vi "Get Ack.vi"(8 "Error In":errorcluster, 11 "connection ID":refnum<k16>) -> (0 "Error Out":errorcluster, 2 "Ack status":bool, 3 "connection ID out":refnum<k16>)   [LabVIEW 2016, in "MKR1000.lvlib"]
doc: "This VI manage the acquisition of the ACK packet. This VI guarantees that the command has been received and managed by MKR1000.\n\nNOTE:\nThe MKR1000 VI Library uses UDP. UDP is a connectionless protocol. With the term \"connection\" is intended that MKR1000 gives back an ACKnoledgment packet for each command sent. If no packet is returned (MKR1000 not connected to the net, out of range, etc.), the command is intended LOST and the VIs attempts to send the command again few times before returning Error 5000"
uses:
  MKR1000.lvlib
  <vilib>/Utility/error.llb/Error Cluster From Error Code.vi
  <vilib>/ErrorRing/Error Ring.xnode
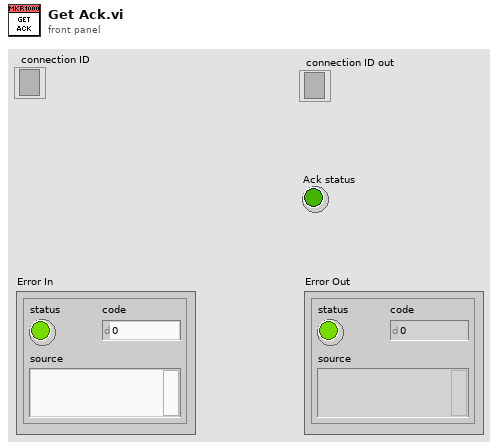
[diagram p1: front panel]
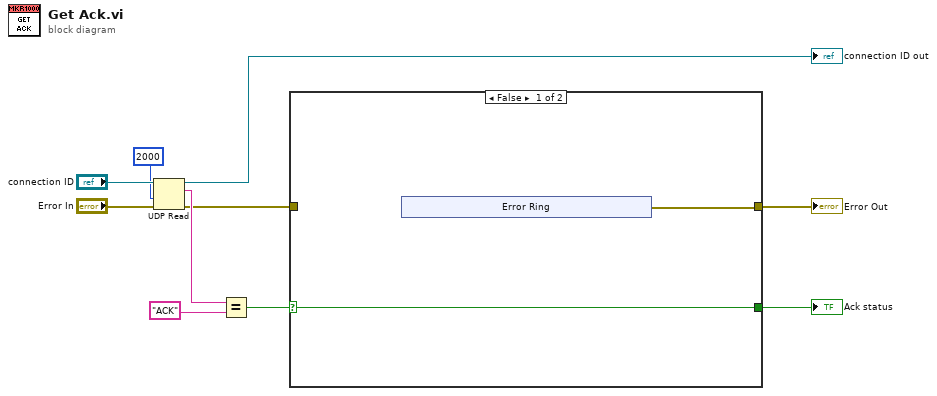
[diagram p0: block diagram]
diagram:
  n1 = UDP Read(connection ID="connection ID", timeout ms (25000)=2000, 8:"Error In") -> (data out=w10:string, error out=w7:errorcluster, 3:→"connection ID out":refnum<k16>)  [unwired: 1 in, 2 out]
  n2 = Equal?(x=w10, y="ACK" ("x")) -> (x = y?=w8:bool)
  n3 = case shown="False" w8 {
    selector: w8 -> [w11 w18]
    tunnel: w7 -> [_ w19]
    tunnel: [w12 w19] -> w3
    tunnel: [w11 w18] -> w2
    frame False {
      n4 = xnode "Error Ring"() -> ("error out"=w12:errorcluster)
    }
    frame True {
    }
  }
  "Error Out" <- w3
  "Ack status" <- w2
